vi "TIO SLIP Serial Read.vi"(8 "error in (no error)":errorcluster, 11 "VISA resource name":refnum<visa-resource-name>) -> (0 "error out":errorcluster, 2 "Payload":string, 3 "VISA resource name 2":refnum<visa-resource-name>)   [LabVIEW 2016]
panel:
  out "CRC32":bool
  out "Raw buffer":string
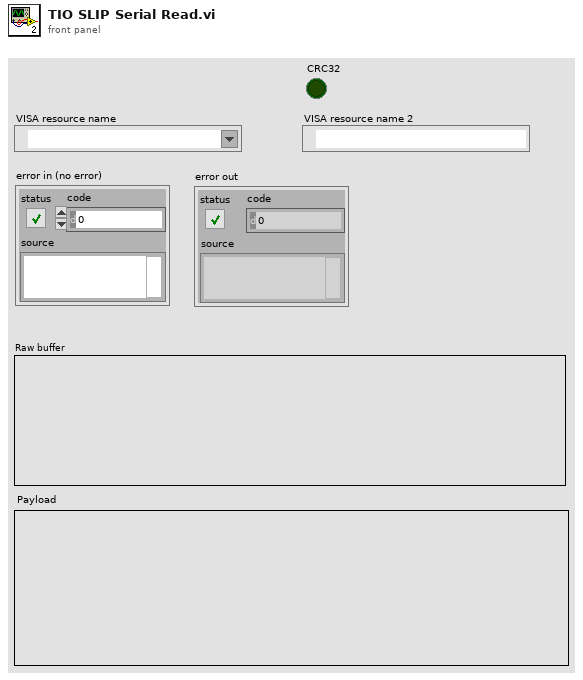
[diagram p1: front panel]
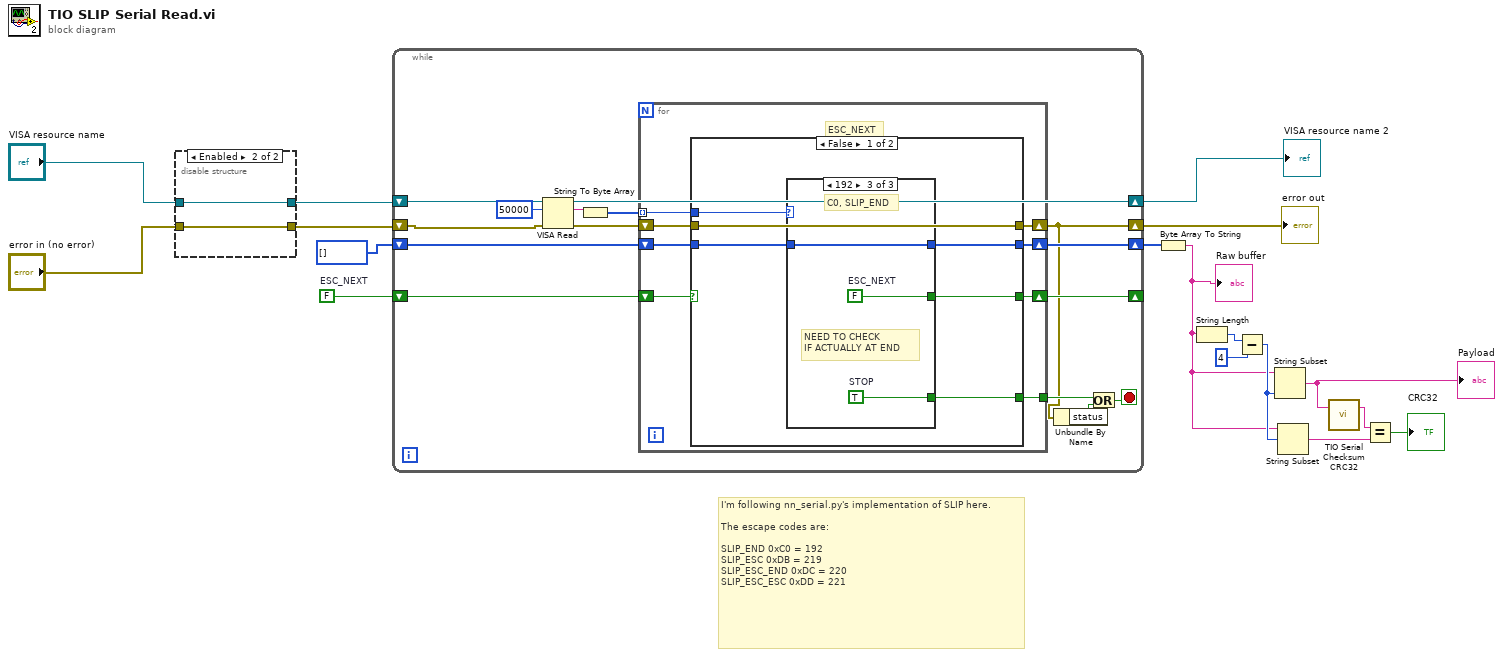
[diagram p0: block diagram]
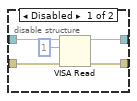
[diagram p2: hidden frame]
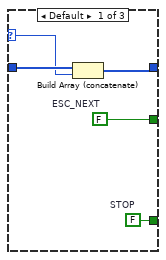
[diagram p3: hidden frame]
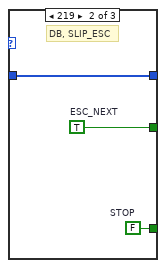
[diagram p4: hidden frame]
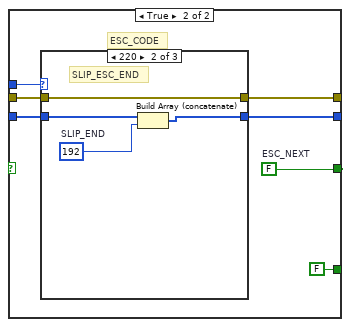
[diagram p5: hidden frame]
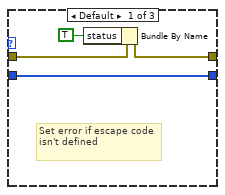
[diagram p6: hidden frame]
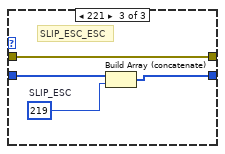
[diagram p7: hidden frame]
diagram:
  w14 = FALSE  # ESC_NEXT
  # "I'm following nn_serial.py's implementation of SLIP here. \n\nThe escape codes are:\n\nSLIP_END\t0xC0 = 192\nSLIP_ESC\t0xDB = 219\nSLIP_ESC_END\t0xDC = 220\nSLIP_ESC_ESC\t0xDD = 221"
  n1 = disable-structure shown="Enabled" {
    disable-tunnel: "VISA resource name" -> [w22 w24]
    disable-tunnel: [w21 w24] -> w11
    disable-tunnel: [w20 w23] -> w10
    disable-tunnel: "error in (no error)" -> [w19 w23]
    frame Disabled {
      n2 = VISA Read(VISA resource name=w22, byte count=u32 1, error in (no error)=w19) -> (VISA resource name out=w21:refnum<visa-resource-name>, error out=w20:errorcluster)  [unwired: 2 out]
    }
    frame Enabled {
    }
  }
  n3 = while {
    shift-right: [w32] -> w13
    shift-left: u8[] [] ("unsigned byte array") -> [w39]
    shift-right: [w37] -> w17
    shift-left: w11 -> [w26]
    shift-right: [w29] -> w16
    shift-left: w10 -> [w25]
    shift-right: [w35] -> _
    shift-left: w14 -> [w38]
    stop <- w30 stop-if-true
    n4 = VISA Read(VISA resource name=w26, byte count=u32 50000, error in (no error)=w25) -> (VISA resource name out=w37:refnum<visa-resource-name>, read buffer=w36:string, error out=w34:errorcluster)  [unwired: 1 out]
    n5 = String To Byte Array(string=w36) -> (unsigned byte array=w33:u8[])
    n6 = for {
      tunnel: [w44] -> w31
      shift-right: [w45] -> w35
      shift-left: w38 -> [w46]
      shift-right: [w42] -> w29
      shift-left: w34 -> [w43]
      tunnel: w33 -> [w41] mode=indexing
      shift-right: [w40] -> w32
      shift-left: w39 -> [w47]
      # "ESC_NEXT"
      n7 = case shown="False" w46 {
        tunnel: w47 -> [w53 w71]
        tunnel: [w52 w70] -> w40
        tunnel: w41 -> [w50 w69]
        tunnel: [w51 w68] -> w45
        tunnel: [w48 w67] -> w42
        tunnel: [w49 FALSE ("STOP")] -> w44
        tunnel: w43 -> [w48 w65]
        frame False {
          n8 = case shown="192" w50 {
            selector: w50 -> [w57 _ _]
            tunnel: w53 -> [w58 w61 w64]
            tunnel: [w56 w61 w64] -> w52
            tunnel: [w55 w60 w63] -> w51
            tunnel: [w54 w59 w62] -> w49
            frame Default {
              w54 = FALSE  # STOP
              w55 = FALSE  # ESC_NEXT
              n9 = Build Array (concatenate)(w58, w57) -> (w56:u8[])
            }
            frame 219 {
              w59 = FALSE  # STOP
              w60 = TRUE  # ESC_NEXT
              # "DB, SLIP_ESC"
            }
            frame 192 {
              w62 = TRUE  # STOP
              w63 = FALSE  # ESC_NEXT
              # "NEED TO CHECK\nIF ACTUALLY AT END"
              # "C0, SLIP_END"
            }
          }
        }
        frame True {
          w68 = FALSE  # ESC_NEXT
          # "ESC_CODE"
          n10 = case shown="220" w69 {
            tunnel: w71 -> [w73 w78 w82]
            tunnel: [w73 w77 w81] -> w70
            tunnel: [w75 w76 w80] -> w67
            tunnel: w65 -> [w72 w76 w80]
            frame Default {
              # "Set error if escape code isn't defined"
              n11 = Bundle By Name(cluster=w72, "status"=TRUE) -> (w75:errorcluster)
            }
            frame 220 {
              w79 = u8 192  # SLIP_END
              # "SLIP_ESC_END"
              n12 = Build Array (concatenate)(w78, w79) -> (w77:u8[])
            }
            frame 221 {
              w83 = u8 219  # SLIP_ESC
              # "SLIP_ESC_ESC"
              n13 = Build Array (concatenate)(w82, w83) -> (w81:u8[])
            }
          }
        }
      }
    }
    n14 = Unbundle By Name(w29) -> ("status"=w28:bool)
    n15 = Or(x=w31, y=w28) -> (x .or. y?=w30:bool)
  }
  "error out" <- w16
  "VISA resource name 2" <- w17
  n16 = Byte Array To String(unsigned byte array=w13) -> (string=w2:string)
  "Raw buffer" <- w2
  n17 = String Length(string=w2) -> (length=w8:i32)
  n18 = Subtract(x=w8, y=4) -> (x-y=w6:i32)
  n19 = String Subset(string=w2, length (rest)=w6) -> (substring=w5:string)  [unwired: 1 in]
  "Payload" <- w5
  n20 = String Subset(string=w2, offset (0)=w6) -> (substring=w1:string)  [unwired: 1 in]
  n21 = call "TIO Serial Checksum CRC32.vi"("String"=w5) -> ("CRC32 Little Endian String"=w4:string)  [unwired: 1 in, 1 out]
  n22 = Equal?(x=w4, y=w1) -> (x = y?=→"CRC32":bool)
